vi "Agilent DSO1000 Series Edge Triggered Acquisition.vi"() -> ()   [LabVIEW 2010]
doc: "This example shows how to configure the oscilloscope to perform an edge-triggered waveform acquisition."
uses:
  <instrlib>/Agilent DSO1000 Series/Public/Configure/Configure Trigger (Edge).vi
  <instrlib>/Agilent DSO1000 Series/Public/Data/Read Waveform (Single).vi
  <instrlib>/Agilent DSO1000 Series/Agilent DSO1000 Series.lvlib
panel:
  in  "Timebase (1E-6 s)":dbl=1e-06
  in  "Probe Attenuation (3: 1X)":u16(ring)=3 items=["0.001X", "0.01X", "0.1X", "1X", "10X", "100X", "1000X"]
  in  "Channel (1: Channel 1)":u16(ring)=1 items=["Channel 1"=1, "Channel 2"=2, "Channel 3"=3, "Channel 4"=4]
  in  "Vertical Coupling (1: DC)":u16(ring)=1 items=["AC", "DC", "Ground"]
  in  "Vertical Range (1.0 V)":dbl=1.0
  in  "Trigger Level (0.0 V)":dbl
  out "Waveform Data":waveform(dbl)(graph)
  in  "VISA resource name":refnum<visa-resource-name>
  # "(c) 2009 National Instruments.  ALL RIGHTS RESERVED."
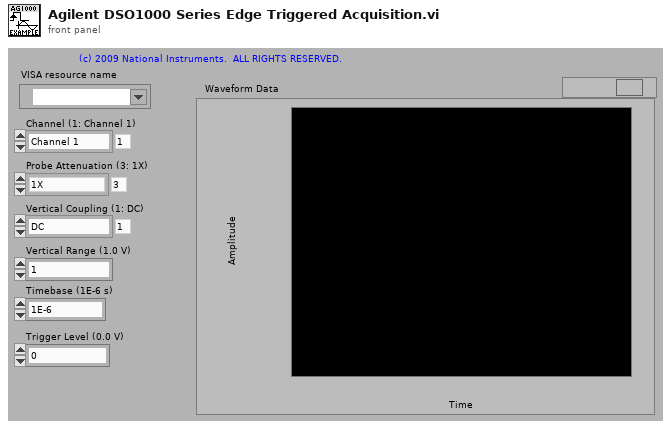
[diagram p1: front panel]
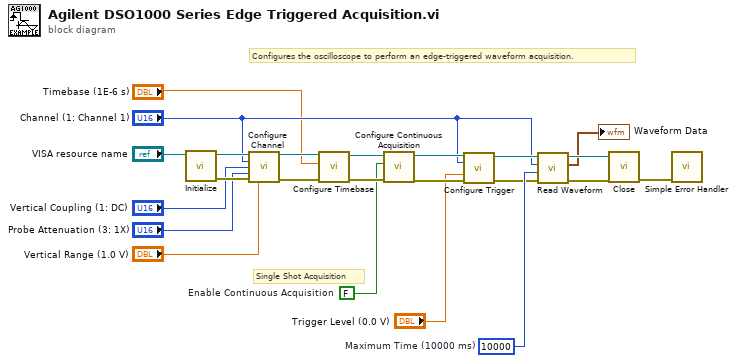
[diagram p0: block diagram]
diagram:
  w5 = u32 10000  # Maximum Time (10000 ms)
  w11 = FALSE  # Enable Continuous Acquisition
  # "Configures the oscilloscope to perform an edge-triggered waveform acquisition."
  # "Single Shot Acquisition"
  n1 = call <instrlib>:"Initialize.vi"("VISA resource name"="VISA resource name") -> ("error out"=w18:errorcluster, "VISA resource name out"=w19:refnum<visa-resource-name>)  [unwired: 9 in]
  n2 = call <instrlib>:"Configure Channel.vi"("VISA resource name"=w19, "Channel (1: Channel 1)"="Channel (1: Channel 1)", "Vertical Coupling (1: DC)"="Vertical Coupling (1: DC)", "Probe Attenuation (3: 1X)"="Probe Attenuation (3: 1X)", "error in (no error)"=w18, "Vertical Range (10.0 V)"="Vertical Range (1.0 V)") -> ("VISA resource name out"=w21:refnum<visa-resource-name>, "error out"=w22:errorcluster)  [unwired: 8 in]
  n3 = call <instrlib>:"Configure Timebase.vi"("error in (no error)"=w22, "Timebase (1E-6 s)"="Timebase (1E-6 s)", "VISA resource name"=w21) -> ("error out"=w14:errorcluster, "VISA resource name out"=w17:refnum<visa-resource-name>)  [unwired: 7 in]
  n4 = call <instrlib>:"Configure Continuous Acquisition.vi"("error in (no error)"=w14, "Enable Continuous Acquisition (T:Enable)"=w11, "VISA resource name"=w17) -> ("error out"=w15:errorcluster, "VISA resource name out"=w16:refnum<visa-resource-name>)  [unwired: 7 in]
  n5 = call-poly <instrlib>:"Configure Trigger.vi"("VISA resource name"=w16, "Trigger Source (1: Channel 1)"="Channel (1: Channel 1)", "Trigger Level (0.0 V)"="Trigger Level (0.0 V)", "error in (no error)"=w15) -> ("VISA resource name out"=w6:refnum<visa-resource-name>, "error out"=w4:errorcluster)  [unwired: 10 in]
  n6 = call-poly <instrlib>:"Read Waveform.vi"("error in (no error)"=w4, "Maximum Time (10000 ms)"=w5, "Channel (1: Channel 1)"="Channel (1: Channel 1)", "VISA resource name"=w6) -> ("error out"=w7:errorcluster, "Waveform Data"=→"Waveform Data":waveform(dbl), "VISA resource name out"=w9:refnum<visa-resource-name>)  [unwired: 5 in]
  n7 = call <instrlib>:"Close.vi"("error in (no error)"=w7, "VISA resource name"=w9) -> ("error out"=w23:errorcluster)  [unwired: 9 in]
  n8 = call <vilib>:"Simple Error Handler.vi"("error in (no error)"=w23) -> ()  [unwired: 4 in, 5 out]
